vi "Run All.vi"(8 "Error In":errorcluster) -> (0 "Error Out":errorcluster)   [LabVIEW 2018, in "Tests.lvlib" / "SFTP Attributes.lvlib"]
uses:
  SFTP Attributes.lvlib
  <vilib>/addons/_JKI Toolkits/Caraya/classes/Test/Test.lvclass
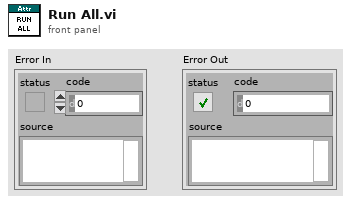
[diagram p1: front panel]
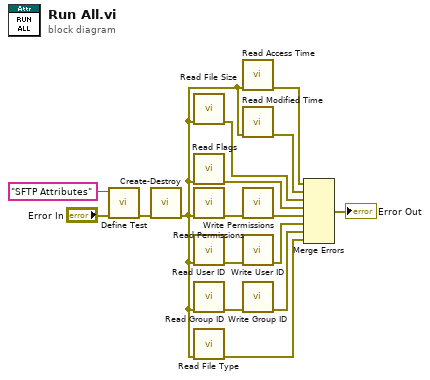
[diagram p0: block diagram]
diagram:
  n1 = call <vilib>:"Define Test.vi"("error in (no error)"="Error In", "Label (VI Title)"="SFTP Attributes") -> ("error out"=w14:errorcluster)  [unwired: 9 in]
  n2 = call "Create-Destroy.vi"("Error In"=w14) -> ("Error Out"=w2:errorcluster)  [unwired: 10 in]
  n3 = call "Read File Size.vi"("Error In"=w2) -> ("Error Out"=w8:errorcluster)  [unwired: 10 in]
  n4 = call "Read Flags.vi"("Error In"=w2) -> ("Error Out"=w7:errorcluster)  [unwired: 10 in]
  n5 = call "Read Permissions.vi"("Error In"=w2) -> ("Error Out"=w13:errorcluster)  [unwired: 10 in]
  n6 = call "Read User ID.vi"("Error In"=w2) -> ("Error Out"=w12:errorcluster)  [unwired: 10 in]
  n7 = call "Read Group ID.vi"("Error In"=w2) -> ("Error Out"=w11:errorcluster)  [unwired: 10 in]
  n8 = call "Read File Type.vi"("Error In"=w2) -> ("Error Out"=w1:errorcluster)  [unwired: 10 in]
  n9 = call "Read Access Time.vi"("Error In"=w2) -> ("Error Out"=w10:errorcluster)  [unwired: 10 in]
  n10 = call "Read Modified Time.vi"("Error In"=w2) -> ("Error Out"=w9:errorcluster)  [unwired: 10 in]
  n11 = call "Write Permissions.vi"("Error In"=w13) -> ("Error Out"=w6:errorcluster)  [unwired: 10 in]
  n12 = call "Write User ID.vi"("Error In"=w12) -> ("Error Out"=w5:errorcluster)  [unwired: 10 in]
  n13 = call "Write Group ID.vi"("Error In"=w11) -> ("Error Out"=w4:errorcluster)  [unwired: 10 in]
  n14 = Merge Errors(w10, w9, w8, w7, w6, w5, w4, w1) -> (→"Error Out":errorcluster)
